vi "backward.vi"(8 "error in (no error)":errorcluster, 11 "Value in":refnum<class "Value.lvclass">) -> (0 "error out":errorcluster, 3 "Value out":refnum<class "Value.lvclass">)   [LabVIEW 2023, in "LabGRAD.lvlib" / "Value.lvclass"]
uses:
  Value.lvclass
panel:
  out "A out":refnum<class "Value.lvclass">[](array[class])
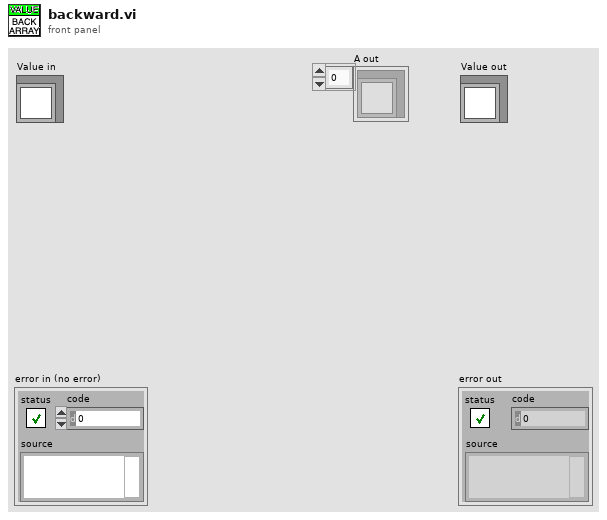
[diagram p1: front panel]
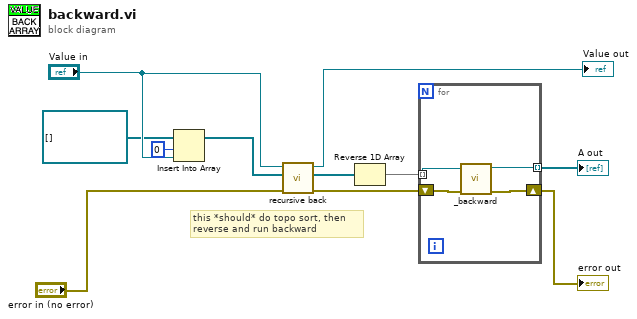
[diagram p0: block diagram]
diagram:
  # "this *should* do topo sort, then \nreverse and run backward"
  n1 = Insert Into Array(array=refnum<class "Value.lvclass">[] [], index=0, new element="Value in") -> (w7:refnum<class "Value.lvclass">[])
  n2 = call "recursive back.vi"("error in (no error)"="error in (no error)", "A in"=w7, "Value in"="Value in") -> ("error out"=w4:errorcluster, "A out"=w5:refnum<class "Value.lvclass">[], "Value out"=→"Value out":refnum<class "Value.lvclass">)  [unwired: 6 in]
  n3 = Reverse 1D Array(array=w5) -> (reversed array=w1:refnum<class "Value.lvclass">[])
  n4 = for {
    tunnel: w1 -> [w15] mode=indexing
    shift-right: [w14] -> w2
    shift-left: w4 -> [w13]
    tunnel: [w12] -> w3 mode=indexing
    n5 = call "_backward.vi"("error in (no error)"=w13, "In"=w15) -> ("error out"=w14:errorcluster, "Out"=w12:refnum<class "Value.lvclass">)  [unwired: 8 in]
  }
  "error out" <- w2
  "A out" <- w3
